vi "dc-rises.vi"(2 "S":bool, 3 "C":bool, 4 "D":bool, 5 "R":bool) -> (0 "notQ":bool, 1 "Q":bool)   [LabVIEW 2013]
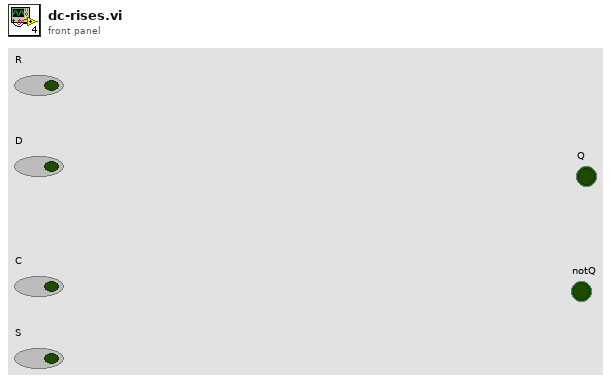
[diagram p1: front panel]
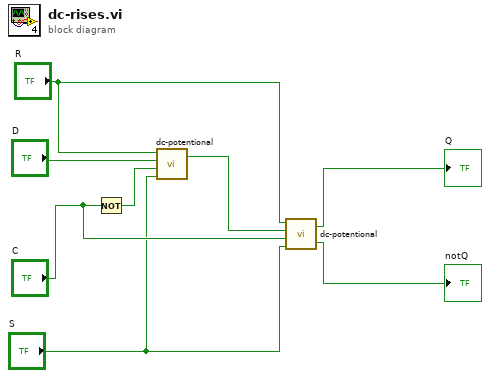
[diagram p0: block diagram]
diagram:
  n1 = Not(x="C") -> (.not. x?=w6:bool)
  n2 = call "dc-potentional.vi"("S"="S", "C"=w6, "D"="D", "R"="R") -> ("Q"=w7:bool)  [unwired: 1 out]
  n3 = call "dc-potentional.vi"("S"="S", "C"="C", "D"=w7, "R"="R") -> ("notQ"=→"notQ":bool, "Q"=→"Q":bool)
